vi "Make Command Node Rectangles.vi"(0 "Icon Rectangle":T2, 6 "Node Rectangle":T2, 8 "Height Padding":dbl, 10 "Width Padding":dbl) -> (14 "New Icon Rectangle":T1, 15 "Text Rectangle":T1)   [LabVIEW 2025]
uses:
  <vilib>/Analysis/baseanly.llb/Mean (DBL).vi
  <vilib>/Analysis/NI_AALBase.lvlib
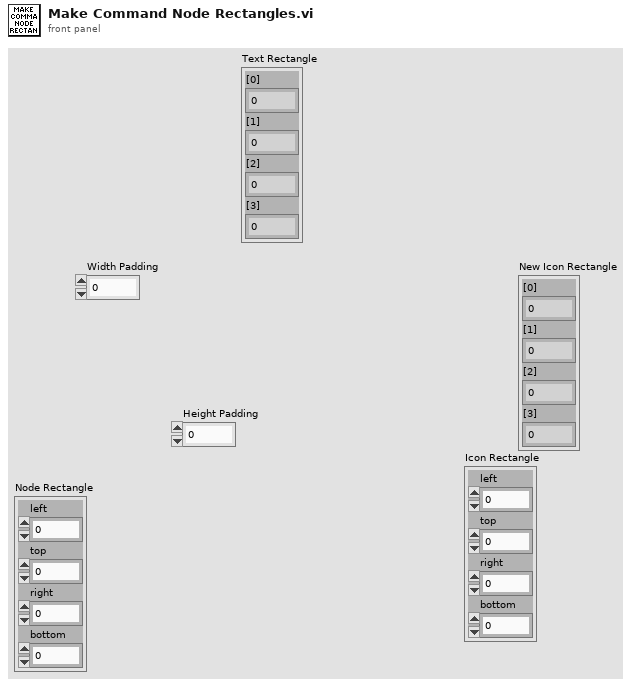
[diagram p1: front panel]
types:
  T1 = cluster{"[0]":dbl, "[1]":dbl, "[2]":dbl, "[3]":dbl}
  T2 = cluster{"left":i16, "top":i16, "right":i16, "bottom":i16}
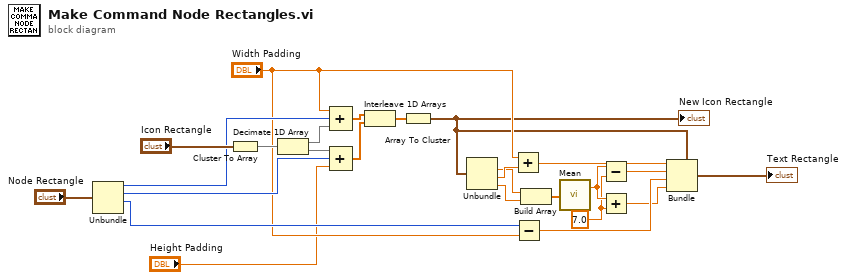
[diagram p0: block diagram]
diagram:
  w4 = 7.0
  n1 = Unbundle("Node Rectangle") -> ("left"=w16:i16, "top"=w17:i16, "right"=w15:i16)  [unwired: 1 out]
  n2 = Cluster To Array(cluster="Icon Rectangle") -> (array=w20:i16[])
  n3 = Decimate 1D Array(w20) -> (w21:i16[], w22:i16[])
  n4 = Compound Arithmetic op=unknown("Width Padding", w16, w21) -> (w23:dbl[])
  n5 = Compound Arithmetic op=unknown(w22, w17, "Height Padding") -> (w24:dbl[])
  n6 = Interleave 1D Arrays(w23, w24) -> (w25:dbl[])
  n7 = Array To Cluster(array=w25) -> (cluster=w13:T1)
  "New Icon Rectangle" <- w13
  n8 = Unbundle(w13) -> ("[1]"=w8:dbl, "[2]"=w10:dbl, "[3]"=w7:dbl)  [unwired: 1 out]
  n9 = Add(x="Width Padding", y=w10) -> (x+y=w12:dbl)
  n10 = Subtract(x=w15, y="Width Padding") -> (x-y=w11:dbl)
  n11 = Build Array(w8, w7) -> (w6:dbl[])
  n12 = call-poly <vilib>:"Mean.vi"("X"=w6) -> ("mean"=w5:dbl)  [unwired: 1 out]
  n13 = Subtract(x=w5, y=w4) -> (x-y=w3:dbl)
  n14 = Add(x=w5, y=w4) -> (x+y=w2:dbl)
  n15 = Bundle(cluster=w13, "[0]"=w12, "[1]"=w3, "[2]"=w11, "[3]"=w2) -> (→"Text Rectangle":T1)
